vi "Writer.vi"(0 "Ethernet MAC - Custom.lvclass":refnum<class "Ethernet MAC - Custom.lvclass">, 7 "niInstr Ethernet MAC Raw Stream v1.lvclass":refnum<class "niInstr Ethernet MAC Raw Stream v1.lvclass">) -> (4 "Ethernet MAC - Custom.lvclass out":refnum<class "Ethernet MAC - Custom.lvclass">, 13 "ready for input?":bool)   [LabVIEW 2020, in "Ethernet MAC - Custom.lvclass"]
uses:
  Ethernet MAC - Custom.lvclass
  <instrlib>/_niInstr/Network/Ethernet/MAC/Raw Stream/v1/niInstr Ethernet MAC Raw Stream v1.lvclass
  <instrlib>/_niInstr/Network/Ethernet/MAC/API/v1/FPGA/niInstr Ethernet MAC v1.lvclass
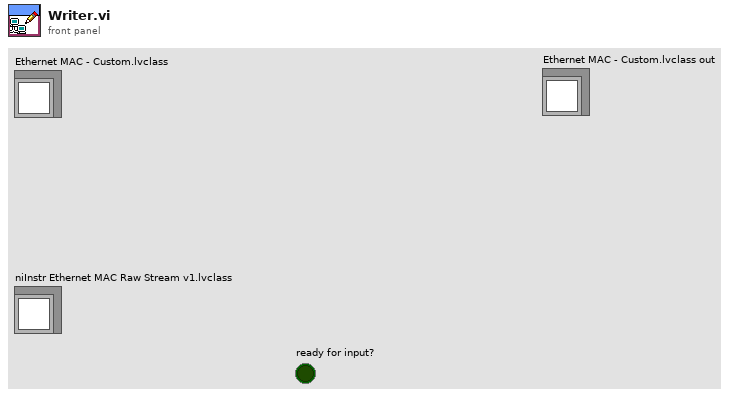
[diagram p1: front panel]
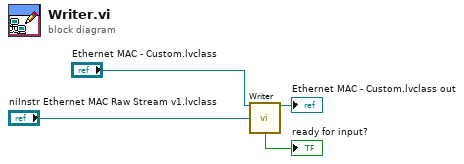
[diagram p0: block diagram]
diagram:
  n1 = call-parent "Writer.vi"("niInstr Ethernet MAC v1.lvclass"="Ethernet MAC - Custom.lvclass", "niInstr Ethernet MAC Raw Stream v1.lvclass"="niInstr Ethernet MAC Raw Stream v1.lvclass") -> ("niInstr Ethernet MAC v1.lvclass out"=→"Ethernet MAC - Custom.lvclass out":refnum<class "Ethernet MAC - Custom.lvclass">, "ready for input?"=→"ready for input?":bool)  [unwired: 12 in]
